vi "PID_c2d.vi"(0 "kp":dbl, 1 "ek":dbl, 5 "ti":dbl, 7 "td":dbl, 9 "Ts":dbl, 12 "u2k-1":dbl, 13 "u1k-1":dbl) -> (6 "uk":dbl, 8 "u1k":dbl, 10 "u2k":dbl)   [LabVIEW 2019]
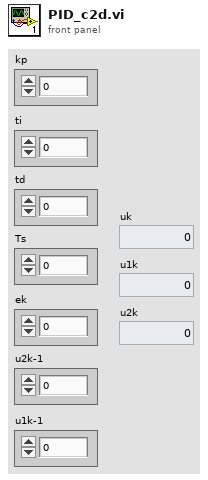
[diagram p1: front panel]
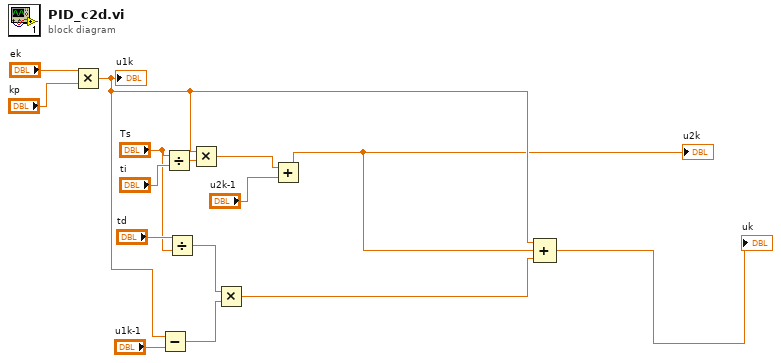
[diagram p0: block diagram]
diagram:
  n1 = Multiply(x="ek", y="kp") -> (x*y=w4:dbl)
  "u1k" <- w4
  n2 = Subtract(x=w4, y="u1k-1") -> (x-y=w5:dbl)
  n3 = Divide(x="Ts", y="ti") -> (x/y=w12:dbl)
  n4 = Divide(x="td", y="Ts") -> (x/y=w6:dbl)
  n5 = Multiply(x=w4, y=w12) -> (x*y=w10:dbl)
  n6 = Multiply(x=w6, y=w5) -> (x*y=w3:dbl)
  n7 = Add(x=w10, y="u2k-1") -> (x+y=w1:dbl)
  "u2k" <- w1
  n8 = Compound Arithmetic op=ADD(w4, w1, w3) -> (→"uk":dbl)
